vi "Calibration Audit v1.vi"() -> ()   [LabVIEW 2014]
doc: "Obtains calibration information for hardware on selected target."
uses:
  <vilib>/Utility/error.llb/DialogType.ctl
  <vilib>/Utility/sysdir.llb/System Directory Type.ctl
  <vilib>/Utility/miscctls.llb/LVRowAndColumnTypeDef.ctl
  <vilib>/Utility/file.llb/Write To Spreadsheet File (string).vi
  <vilib>/nisyscfg/Close (Hardware).vi
  <vilib>/nisyscfg/Close (System).vi
  <vilib>/nisyscfg/Close (Filter).vi
  <vilib>/nisyscfg/nisyscfg.lvlib
  <resource>/objmgr/nisysapi.rc
panel:
  in  "Cal File Destination":path
  in  "START":bool
  in  "User Name":string
  in  "Password":string
  in  "Target (localhost)":refnum<k21>="localhost"
  out "Calibration Results":string[][](table)
  # "Overview: Obtains calibration information for the hardware on a selected target.\nRequirements: NI System Configuration, applicable device drivers\nInstructions:\n1. Select Target. Enter User Name and Password if necessary. \n2. Select a destination for your calibration file, or leave as default to save to desktop.\n***This program will automatically overwrite a file of the same name if it exists at that destination.***\n3. Click the START button.\nThe recommended next calibration date does not account for shelf life. Visit ni.com/calibration to generate an official copy of your NI calibration certificate.\n***If you receive an error about the System Configuration API, make sure your RT target is not in Safe Mode***"
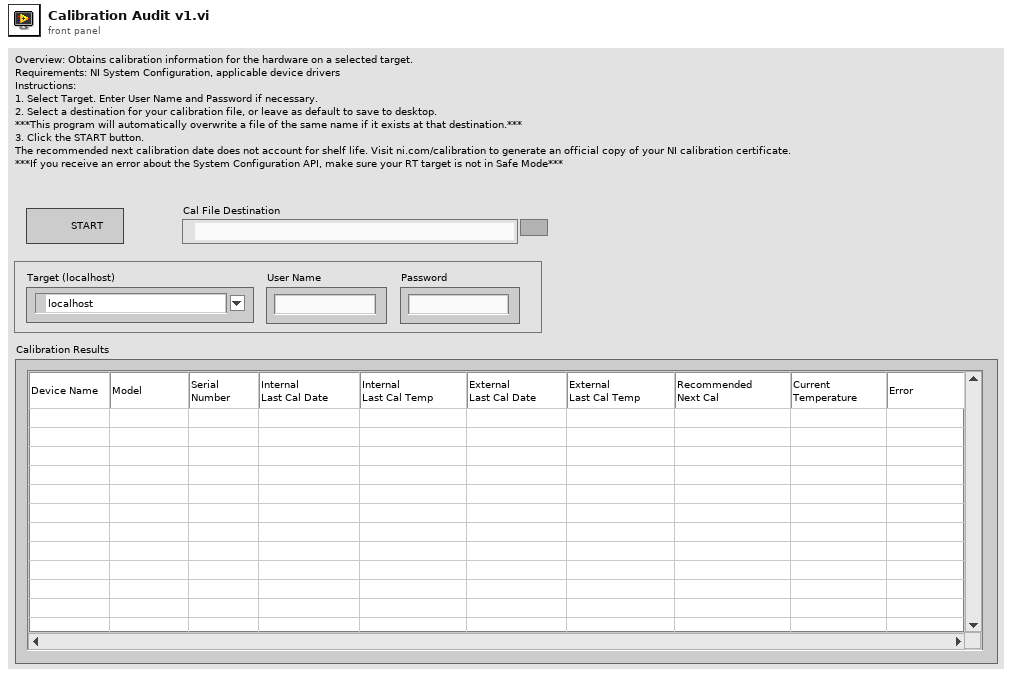
[diagram p1: front panel]
types:
  T1 = typedef "System Directory Type.ctl" = i32
  T2 = typedef "DialogType.ctl" = u16
  T3 = typedef "LVRowAndColumnTypeDef.ctl" = cluster{"Row":i32, "Column":i32}
  T4 = cluster{"Last Calibrated":timestamp, "Last Temperature":dbl, "Recommended Next Calibration":timestamp}
  T5 = cluster{"Last Calibrated":timestamp, "Last Temperature":dbl}
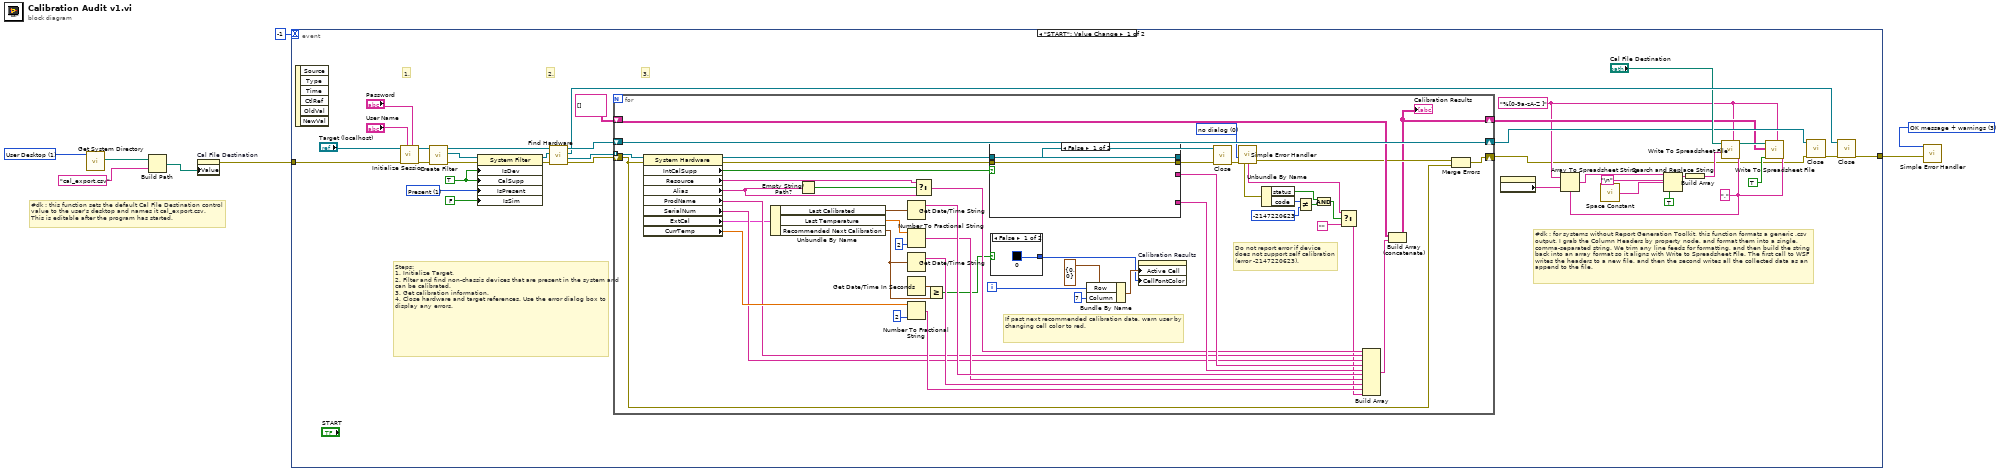
[diagram p0: block diagram]
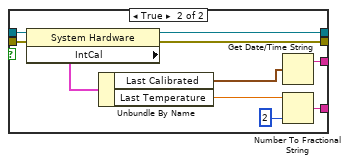
[diagram p2: hidden frame]
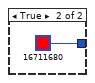
[diagram p3: hidden frame]
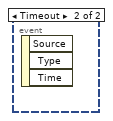
[diagram p4: hidden frame]
diagram:
  w3 = T1 1 items=["User Home"=0, "User Desktop"=1, "User Documents"=2, "User Application Data"=3, "User Preferences"=4, "User Temporary"=5, "Public Documents"=6, "Public Application Data"=7, "Public Preferences"=8, "Public Cache"=13, "System Core Libraries"=9, "System Installed Libraries"=10, "Application Files"=11, "Boot Volume Root"=12] ("system directory type")
  w7 = T2 3 items=["no dialog", "OK message", "continue or stop message", "OK message + warnings", "continue/stop + warnings"] ("type of dialog (OK msg:1)")
  # "#dk : this function sets the default Cal File Destination control\nvalue to the user's desktop and names it cal_export.csv. \nThis is editable after the program has started."
  n1 = call <vilib>:"Get System Directory.vi"("system directory type"=w3) -> ("system directory"=w1:path)  [unwired: 10 in]
  n2 = Build Path(base path=w1, name or relative path="cal_export.csv") -> (appended path=w5:path)
  n3 = property on="Cal File Destination" class="Path"("Value"=w5) -> (error out=w4:errorcluster)  [unwired: 2 in, 1 out]
  n4 = event shown="[0] \"START\": Value Change" {
    selector: _ -> [_ _]
    dyn-events: _ -> [_ _]
    timeout: -1 -> [_ _]
    tunnel: [w25 _] -> w8
    tunnel: w4 -> [w24 _]
    event "START": Value Change {
      w17 = "%[0-9a-zA-Z ]" ("format (%s)")
      w16 = "," ("delimiter (\\t)")
      w35 = 1 items=["Unknown"=-1, "Not Present"=0, "Present"=1] ("Is Present")
      w42 = TRUE ("Is Device")
      # "#dk : for systems without Report Generation Toolkit, this function formats a generic .csv\noutput. I grab the Column Headers by property node, and format them into a single,\ncomma-separated string. We trim any line feeds for formatting, and then build the string\nback into an array format so it aligns with Write to Spreadsheet File. The first call to WSF\nwrites the headers to a new file, and then the second writes all the collected data as an \nappend to the file."
      # "3."
      # "2."
      # "1."
      # "Steps:\n1. Initialize Target.\n2. Filter and find non-chassis devices that are present in the system and can be calibrated.\n3. Get calibration information.\n4. Close hardware and target references. Use the error dialog box to display any errors."
      n5 = event-data() -> ()  [unwired: 1 in, 6 out]
      n6 = call <vilib>:"Initialize Session.vi"("Password"="Password", "User Name"="User Name", "error in (no error)"=w24, "Target (localhost)"="Target (localhost)") -> ("error out"=w30:errorcluster, "Session out"=w29:refnum<k21>)  [unwired: 6 in]
      n7 = call <vilib>:"Create Filter.vi"("error in (no error)"=w30, "Session in"=w29) -> ("error out"=w43:errorcluster, "Filter out"=w44:refnum<k20>, "Session out"=w39:refnum<k21>)  [unwired: 7 in]
      n8 = property class="System Filter"(reference=w44, error in=w43, "IsDev"=w42, "CalSupp"=w42, "IsPresent"=w35, "IsSim"=FALSE ("Is Simulated")) -> (reference out=w40:refnum<k20>, error out=w41:errorcluster)
      n9 = call <vilib>:"Find Hardware.vi"("error in (no error)"=w41, "Filter in"=w40, "Session in"=w39) -> ("error out"=w31:errorcluster, "Resources out"=w37:refnum<k20>[], "Filter out"=w32:refnum<k20>, "Session out"=w38:refnum<k21>)  [unwired: 1 in, 4 out]
      n10 = for {
        tunnel: w37 -> [w90] mode=indexing
        shift-right: [w45] -> w20
        shift-left: string[][] [] ("appended array") -> [w89]
        shift-right: [w92] -> w22
        shift-left: w38 -> [w92]
        shift-right: [w47] -> w9
        shift-left: w31 -> [w48]
        i -> [w68]
        w67 = T2 0 items=["no dialog", "OK message", "continue or stop message", "OK message + warnings", "continue/stop + warnings"] ("type of dialog (OK msg:1)")
        # "If past next recommended calibration date, warn user by \nchanging cell color to red."
        # "Do not report error if device \ndoes not support self calibration\n(error -2147220623)."
        n11 = property class="System Hardware"(reference=w90, error in=w48) -> (reference out=w55:refnum<k20>, error out=w62:errorcluster, "IntCalSupp"=w56:bool, "Resource"=w57:string, "Alias"=w58:string, "ProdName"=w76:string, "SerialNum"=w75:string, "ExtCal"=w66:T4, "CurrTemp"=w83:dbl)
        n12 = Unbundle By Name(w66) -> ("Last Calibrated"=w60:timestamp, "Last Temperature"=w85:dbl, "Recommended Next Calibration"=w59:timestamp)
        n13 = Empty String/Path?(string/path=w58) -> (empty?=w91:bool)
        n14 = Get Date/Time String(seconds (now)=w60) -> (date string=w80:string)  [unwired: 2 in, 1 out]
        n15 = Number To Fractional String(number=w85, precision (6)=i16 2) -> (F-format string=w79:string)  [unwired: 2 in]
        n16 = Get Date/Time String(seconds (now)=w59) -> (date string=w78:string)  [unwired: 2 in, 1 out]
        n17 = Get Date/Time In Seconds() -> (seconds since 1Jan1904=w69:timestamp)
        n18 = Number To Fractional String(number=w83, precision (6)=i16 2) -> (F-format string=w82:string)  [unwired: 2 in]
        n19 = Select(t=w57, s=w91, f=w58) -> (s? t:f=w77:string)
        n20 = Greater Or Equal?(x=w69, y=w59) -> (x >= y?=w71:bool)
        n21 = case shown="False" w56 {
          tunnel: [_ w104] -> w87
          tunnel: [_ w103] -> w86
          tunnel: [w93 w99] -> w63
          tunnel: w62 -> [w94 w98]
          tunnel: [w94 w97] -> w61
          tunnel: w55 -> [w93 w95]
          frame False {
          }
          frame True {
            n22 = property class="System Hardware"(reference=w95, error in=w98) -> (reference out=w99:refnum<k20>, error out=w97:errorcluster, "IntCal"=w96:T5)
            n23 = Unbundle By Name(w96) -> ("Last Calibrated"=w101:timestamp, "Last Temperature"=w100:dbl)
            n24 = Get Date/Time String(seconds (now)=w101) -> (date string=w104:string)  [unwired: 2 in, 1 out]
            n25 = Number To Fractional String(number=w100, precision (6)=i16 2) -> (F-format string=w103:string)  [unwired: 2 in]
          }
        }
        n26 = case shown="False" w71 {
          tunnel: [u32 0 u32 16711680] -> w72
          frame False {
          }
          frame True {
          }
        }
        n27 = Bundle By Name(cluster=T3 {"Row"=0, "Column"=0} ("Active Cell:Active Cell"), "Row"=w68, "Column"=7) -> (w73:T3)
        n28 = property on="Calibration Results" class="Tbl (strict)"("Active Cell"=w73, "CellFontColor"=w72) -> ()  [unwired: 2 in, 2 out]
        n29 = call-poly <vilib>:"Close.vi"("error in (no error)"=w61, "Resource in"=w63) -> ("error out"=w49:errorcluster)  [unwired: 9 in]
        n30 = call <vilib>:"Simple Error Handler.vi"("type of dialog (OK msg:1)"=w67, "error in (no error)"=w49) -> ("message"=w65:string)  [unwired: 3 in, 4 out]
        n31 = Unbundle By Name(w49) -> ("status"=w53:bool, "code"=w51:i32)
        n32 = Not Equal?(x=w51, y=-2147220623) -> (x != y?=w52:bool)
        n33 = And(x=w53, y=w52) -> (x .and. y?=w54:bool)
        n34 = Select(t=w65, s=w54, f="") -> (s? t:f=w46:string)
        n35 = Build Array(w77, w76, w75, w87, w86, w80, w79, w78, w82, w46) -> (w88:string[])
        n36 = Build Array (concatenate)(w89, w88) -> (w45:string[][])
        "Calibration Results" <- w45
        n37 = Merge Errors(w49, w48) -> (w47:errorcluster)
      }
      n38 = property on="Calibration Results" class="Tbl (strict)"() -> ("Column Headers[]"=w18:string[])  [unwired: 2 in, 2 out]
      n39 = Array To Spreadsheet String(delimiter (Tab)=w16, array=w18, 3:w17) -> (spreadsheet string=w14:string)
      n40 = call <vilib>:"Space Constant.vi"() -> ("String"=w11:string)
      n41 = Search and Replace String(replace all?=TRUE ("replace all? (F)"), input string=w14, search string="\n", replace string=w11) -> (result string=w15:string)  [unwired: 4 in, 3 out]
      n42 = Build Array(w15) -> (w10:string[])
      n43 = call-poly <vilib>:"Write To Spreadsheet File.vi"("delimiter (\\t)"=w16, "format (%s)"=w17, "1D data"=w10, "file path (dialog if empty)"="Cal File Destination") -> ("new file path (Not A Path if cancelled)"=w21:path)  [unwired: 4 in]
      n44 = call-poly <vilib>:"Write To Spreadsheet File.vi"("delimiter (\\t)"=w16, "format (%s)"=w17, "append to file? (new file:F)"=TRUE, "2D data"=w20, "file path (dialog if empty)"=w21) -> ()  [unwired: 3 in, 1 out]
      n45 = call-poly <vilib>:"Close.vi"("error in (no error)"=w9, "Session in"=w22) -> ("error out"=w33:errorcluster)  [unwired: 9 in]
      n46 = call-poly <vilib>:"Close.vi"("error in (no error)"=w33, "Filter in"=w32) -> ("error out"=w25:errorcluster)  [unwired: 9 in]
    }
    event Timeout {
      n47 = event-data() -> ()  [unwired: 1 in, 3 out]
    }
  }
  n48 = call <vilib>:"Simple Error Handler.vi"("type of dialog (OK msg:1)"=w7, "error in (no error)"=w8) -> ()  [unwired: 3 in, 5 out]
